vi "FTW-SQLite-RandomBLOB.vi"(0 "Number of Bytes":i32=1024, 11 "error in":errorcluster) -> (4 "Random BLOB":string, 15 "error out":errorcluster)   [LabVIEW 2014]
uses:
  error/FTW-ERR-ThrowGenericError.vi
  error/FTW-ERR-ThrowError.vi
  error/FTW-ERR-NoErrorConstant.vi
  error/FTW-ERR-CallChain.vi
  string/FTW-STR-ReplaceWhitespace.vi
panel:
  # "Inputs"
  # "Outputs"
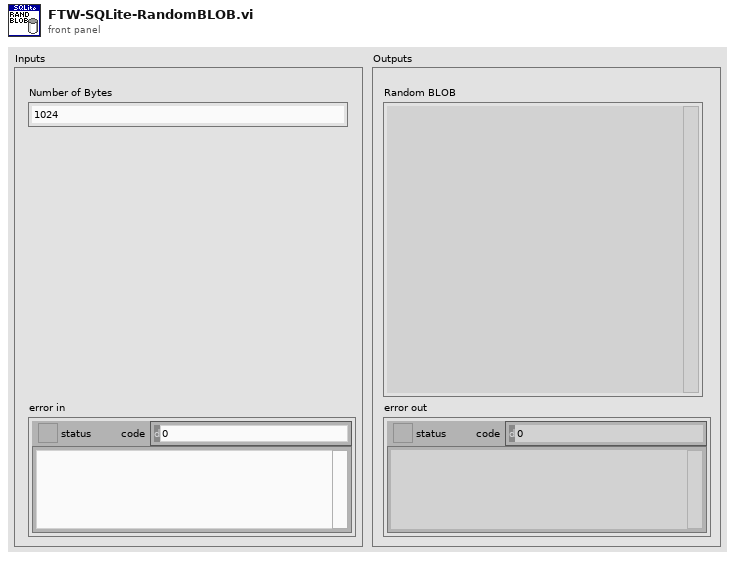
[diagram p1: front panel]
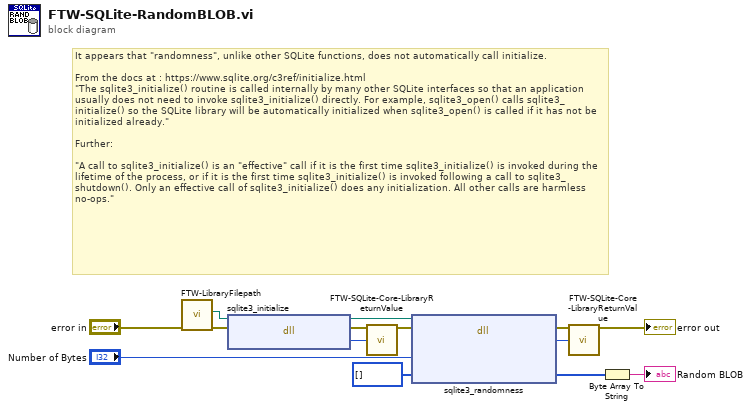
[diagram p0: block diagram]
diagram:
  # "It appears that \"randomness\", unlike other SQLite functions, does not automatically call initialize.\n\nFrom the docs at : https://www.sqlite.org/c3ref/initialize.html\n\"The sqlite3_initialize() routine is called internally by many other SQLite interfaces so that an application usually does not need to invoke sqlite3_initialize() directly. For example, sqlite3_open() calls sqlite3_initialize() so the SQLite library will be automatically initialized when sqlite3_open() is called if it has not be initialized already.\"\n\nFurther:\n\n\"A call to sqlite3_initialize() is an \"effective\" call if it is the first time sqlite3_initialize() is invoked during the lifetime of the process, or if it is the first time sqlite3_initialize() is invoked following a call to sqlite3_shutdown(). Only an effective call of sqlite3_initialize() does any initialization. All other calls are harmless no-ops.\""
  n1 = call "FTW-LibraryFilepath.vi"("error in"="error in") -> ("error out"=w6:errorcluster, "Library Filepath"=w7:path)  [unwired: 8 in, 1 out]
  n2 = dll-call lib="?" fn="sqlite3_initialize"(path in=w7, error in=w6) -> (path out=w3:path, error out=w5:errorcluster, "Return Value"=w4:i32)  [unwired: 1 in]
  n3 = call "FTW-SQLite-Core-LibraryReturnValue.vi"("error in"=w5, "Return Value"=w4) -> ("error out"=w2:errorcluster)  [unwired: 13 in]
  n4 = dll-call lib="?" fn="sqlite3_randomness"(path in=w3, error in=w2, "Number of Bytes"="Number of Bytes", "Random Bytes Buffer"=u8[] []) -> (error out=w13:errorcluster, "Return Value"=w11:i32, "Random Bytes Buffer"=w9:u8[])  [unwired: 2 in, 1 out]
  n5 = call "FTW-SQLite-Core-LibraryReturnValue.vi"("error in"=w13, "Return Value"=w11) -> ("error out"=→"error out":errorcluster)  [unwired: 13 in]
  n6 = Byte Array To String(unsigned byte array=w9) -> (string=→"Random BLOB":string)
